vi "triangle scan.vi"(11 "scan specification":T1) -> (2 "scan locations":u32[](array[numeric]), 3 "scan specification out":T1)   [LabVIEW 2010]
uses:
  scan_specification_tagResonant.ctl
  <vilib>/Analysis/NI_AALBase.lvlib
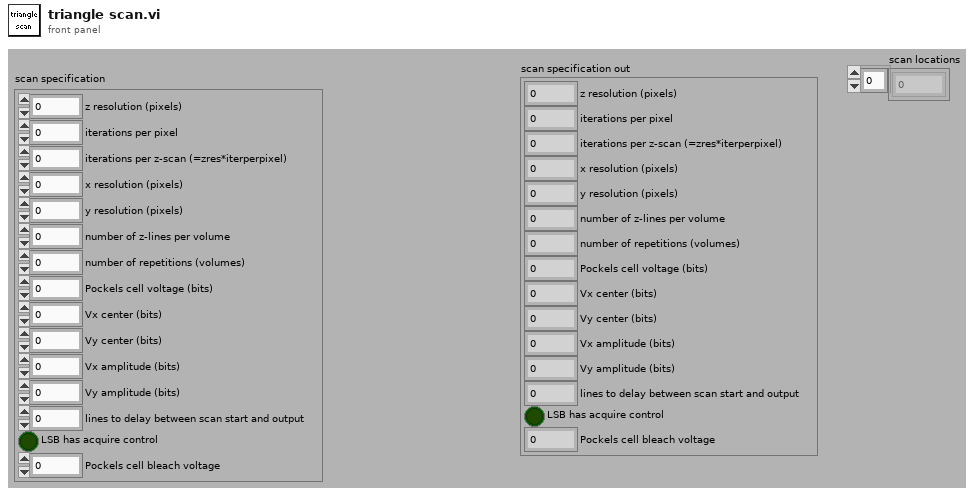
[diagram p1: front panel]
types:
  T1 = typedef "scan_specification_tagResonant.ctl" = cluster{"z resolution (pixels)":u16, "iterations per pixel":u16, "iterations per z-scan (=zres*iterperpixel)":u16, "x resolution (pixels)":u16, "y resolution (pixels)":u16, "number of z-lines per volume":u16, "number of repetitions (volumes)":i32, "Pockels cell voltage (bits)":i16, "Vx center (bits)":i16, "Vy center (bits)":i16, "Vx amplitude (bits)":i16, "Vy amplitude (bits)":i16, "lines to delay between scan start and output":u16, "LSB has acquire control":bool, "Pockels cell bleach voltage":i16}
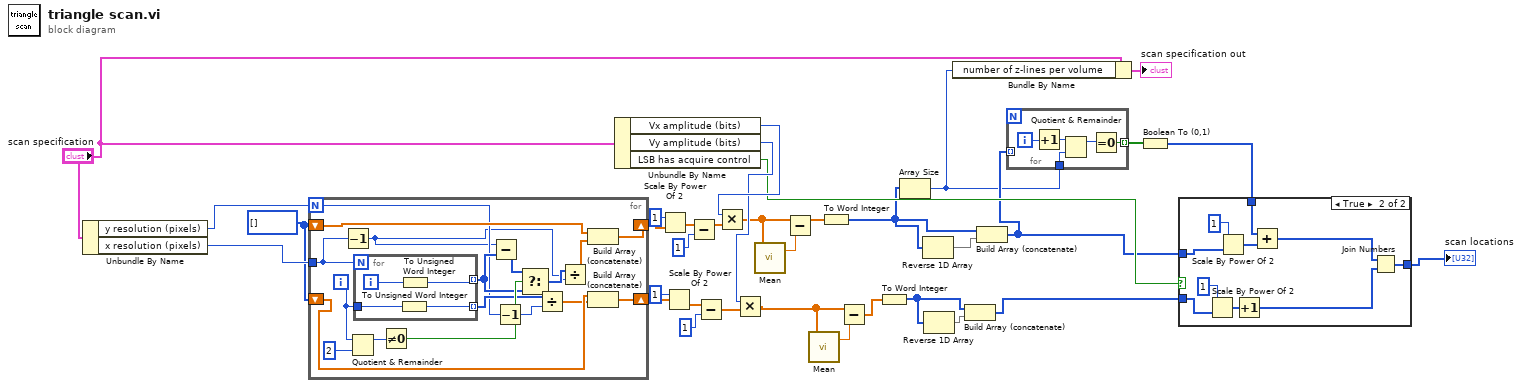
[diagram p0: block diagram]
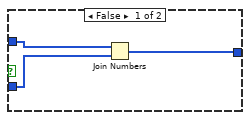
[diagram p2: hidden frame]
diagram:
  w32 = u16[] []
  n1 = Unbundle By Name("scan specification") -> ("y resolution (pixels)"=w33:u16, "x resolution (pixels)"=w34:u16)
  n2 = for {
    N: w33 -> [w37]
    tunnel: w34 -> [w40]
    shift-right: [w46] -> w31
    shift-left: w32 -> [w45]
    shift-right: [w44] -> w21
    shift-left: w32 -> [w43]
    i -> [w52]
    n3 = Decrement(x=w40) -> (x-1=w36:u16)
    n4 = Quotient & Remainder(x=w52, y=2) -> (x-y*floor(x/y)=w50:i32)  [unwired: 1 out]
    n5 = for {
      N: w40 -> [_]
      tunnel: [w54] -> w47 mode=indexing
      tunnel: w52 -> [w55]
      tunnel: [w53] -> w38 mode=indexing
      i -> [w56]
      n6 = To Unsigned Word Integer(number=w55) -> (unsigned 16bit integer=w53:u16)
      n7 = To Unsigned Word Integer(number=w56) -> (unsigned 16bit integer=w54:u16)
    }
    n8 = Not Equal To 0?(x=w50) -> (x != 0?=w49:bool)
    n9 = Subtract(x=w36, y=w47) -> (x-y=w48:u16[])
    n10 = Decrement(x=w37) -> (x-1=w35:i32)
    n11 = Select(t=w48, s=w49, f=w47) -> (s? t:f=w41:u16[])
    n12 = Divide(x=w38, y=w35) -> (x/y=w39:dbl[])
    n13 = Divide(x=w41, y=w36) -> (x/y=w42:dbl[])
    n14 = Build Array (concatenate)(w45, w42) -> (w46:dbl[])
    n15 = Build Array (concatenate)(w43, w39) -> (w44:dbl[])
  }
  n16 = Unbundle By Name("scan specification") -> ("Vx amplitude (bits)"=w30:i16, "Vy amplitude (bits)"=w24:i16, "LSB has acquire control"=w23:bool)
  n17 = Scale By Power Of 2(n=1, x=w31) -> (x*2^n=w20:dbl[])
  n18 = Scale By Power Of 2(n=1, x=w21) -> (x*2^n=w18:dbl[])
  n19 = Subtract(x=w20, y=1) -> (x-y=w28:dbl[])
  n20 = Subtract(x=w18, y=1) -> (x-y=w25:dbl[])
  n21 = Multiply(x=w30, y=w28) -> (x*y=w15:dbl[])
  n22 = Multiply(x=w24, y=w25) -> (x*y=w12:dbl[])
  n23 = call <vilib>:"Mean.vi"("X"=w15) -> ("mean"=w14:dbl)  [unwired: 1 out]
  n24 = Subtract(x=w15, y=w14) -> (x-y=w16:dbl[])
  n25 = call <vilib>:"Mean.vi"("X"=w12) -> ("mean"=w13:dbl)  [unwired: 1 out]
  n26 = To Word Integer(number=w16) -> (16bit integer=w9:i16[])
  n27 = Subtract(x=w12, y=w13) -> (x-y=w11:dbl[])
  n28 = To Word Integer(number=w11) -> (16bit integer=w7:i16[])
  n29 = Array Size(array=w9) -> (size(s)=w4:i32)
  n30 = Reverse 1D Array(array=w9) -> (reversed array=w10:i16[])
  n31 = Reverse 1D Array(array=w7) -> (reversed array=w8:i16[])
  n32 = Bundle By Name(cluster="scan specification", "number of z-lines per volume"=w4) -> (→"scan specification out":T1)
  n33 = Build Array (concatenate)(w7, w8) -> (w6:i16[])
  n34 = Build Array (concatenate)(w9, w10) -> (w5:i16[])
  n35 = for {
    tunnel: w5 -> [_] mode=indexing
    tunnel: w4 -> [w59]
    tunnel: [w57] -> w3 mode=indexing
    i -> [w61]
    n36 = Increment(x=w61) -> (x+1=w60:i32)
    n37 = Quotient & Remainder(x=w60, y=w59) -> (x-y*floor(x/y)=w58:i32)  [unwired: 1 out]
    n38 = Equal To 0?(x=w58) -> (x = 0?=w57:bool)
  }
  n39 = Boolean To (0,1)(Boolean=w3) -> (0, 1=w2:i16[])
  n40 = case shown="True" w23 {
    tunnel: w5 -> [w64 w70]
    tunnel: w6 -> [w63 w74]
    tunnel: [w62 w68] -> w1
    tunnel: w2 -> [_ w66]
    frame False {
      n41 = Join Numbers(hi=w64, lo=w63) -> ((hi.lo)=w62:u32[])
    }
    frame True {
      n42 = Scale By Power Of 2(n=1, x=w74) -> (x*2^n=w72:i16[])
      n43 = Scale By Power Of 2(n=1, x=w70) -> (x*2^n=w67:i16[])
      n44 = Increment(x=w72) -> (x+1=w69:i16[])
      n45 = Add(x=w66, y=w67) -> (x+y=w65:i16[])
      n46 = Join Numbers(hi=w65, lo=w69) -> ((hi.lo)=w68:u32[])
    }
  }
  "scan locations" <- w1
